vi "Untitled 2.vi"() -> ()   [LabVIEW 2017]
panel:
  out "String":string
  out "Boolean 2":bool
  out "Boolean":bool
  in  "Tank":dbl(slide) scale=0.0..10.0
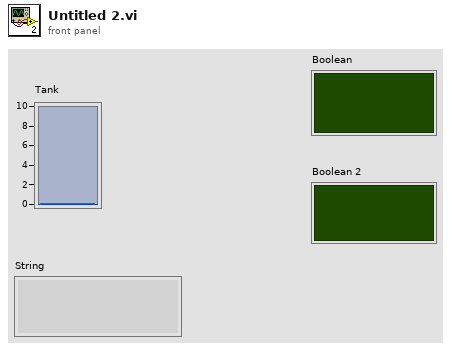
[diagram p1: front panel]
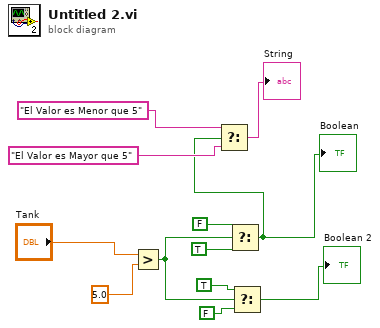
[diagram p0: block diagram]
diagram:
  n1 = Greater?(x="Tank", y=5.0) -> (0:w10:bool)
  n2 = Select(t=FALSE, s=w10, f=TRUE) -> (s? t:f=w3:bool)
  "Boolean" <- w3
  n3 = Select(t="El Valor es Menor que 5", s=w3, f="El Valor es Mayor que 5") -> (s? t:f=→"String":string)
  n4 = Select(t=TRUE, s=w10, f=FALSE) -> (s? t:f=→"Boolean 2":bool)
